vi "examen.vi"() -> ()   [LabVIEW 2016]
uses:
  <vilib>/Utility/file.llb/Write Delimited Spreadsheet (DBL).vi
panel:
  out "rango":bool
  out "supera el maximo":dbl
  out "on/off":bool
  out "valor actual":dbl
  out "Waveform Chart":dbl[][](graph)
  in  "finalizar":bool
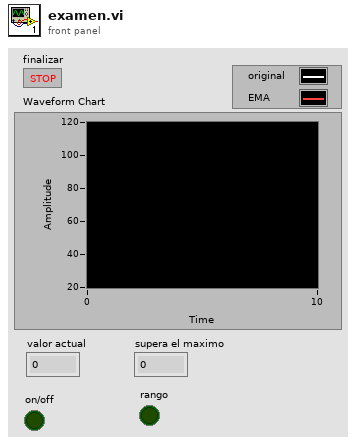
[diagram p1: front panel]
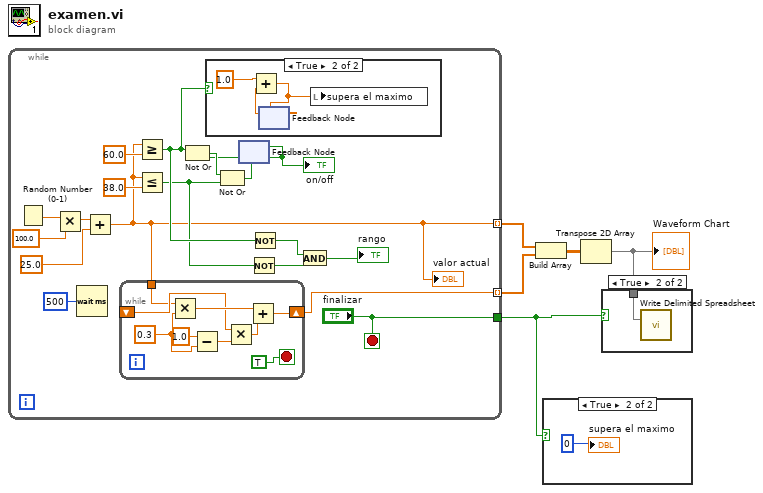
[diagram p0: block diagram]
diagram:
  n1 = while {
    tunnel: [w6] -> w5 mode=indexing
    tunnel: [w7] -> w4 mode=indexing
    tunnel: ["finalizar"] -> w1
    stop <- "finalizar" stop-if-true
    n2 = Random Number (0-1)() -> (number: 0 to 1=w22:dbl)
    n3 = Multiply(x=w22, y=100.0) -> (x*y=w20:dbl)
    n4 = Wait (ms)(milliseconds to wait=u32 500) -> ()  [unwired: 1 out]
    n5 = Add(x=w20, y=25.0) -> (x+y=w6:dbl)
    "valor actual" <- w6
    n6 = while {
      shift-right: [w29] -> w7
      shift-left: _ -> [w30]
      tunnel: w6 -> [w27]
      stop <- TRUE stop-if-true
      w33 = 0.3 ("y")
      n7 = Multiply(x=w27, y=w33) -> (x*y=w31:dbl)
      n8 = Subtract(x=1.0, y=w33) -> (x-y=w34:dbl)
      n9 = Multiply(x=w30, y=w34) -> (x*y=w35:dbl)
      n10 = Add(x=w31, y=w35) -> (x+y=w29:dbl)
    }
    n11 = Greater Or Equal?(x=w6, y=60.0) -> (x >= y?=w13:bool)
    n12 = Less Or Equal?(x=w6, y=38.0) -> (x <= y?=w12:bool)
    n13 = case shown="True" w13 {
      frame False {
      }
      frame True {
        n14 = feedback #1() -> (w25:dbl)  [unwired: 1 in]
        n15 = Add(x=1.0, y=w25) -> (x+y=w24:dbl)
        n16 = feedback-in #1(w24) -> ()
        n17 = local write "supera el maximo"(w24) -> ()
      }
    }
    n18 = feedback #2() -> (w14:bool)  [unwired: 1 in]
    "on/off" <- w14
    n19 = Not Or(1:w14, 2:w13) -> (0:w16:bool)
    n20 = Not Or(1:w12, 2:w16) -> (0:w15:bool)
    n21 = feedback-in #2(w15) -> ()
    n22 = Not(x=w12) -> (.not. x?=w10:bool)
    n23 = Not(x=w13) -> (.not. x?=w11:bool)
    n24 = And(x=w11, y=w10) -> (x .and. y?=→"rango":bool)
  }
  n25 = Build Array(w5, w4) -> (w3:dbl[][])
  n26 = case shown="True" w1 {
    frame False {
    }
    frame True {
      "supera el maximo" <- 0
    }
  }
  n27 = Transpose 2D Array(2D array=w3) -> (transposed array=w2:dbl[][])
  "Waveform Chart" <- w2
  n28 = case shown="True" w1 {
    tunnel: w2 -> [_ w37]
    frame False {
    }
    frame True {
      n29 = call-poly <vilib>:"Write Delimited Spreadsheet.vi"("2D data"=w37) -> ()  [unwired: 13 in, 2 out]
    }
  }
